vi "Set IConfiguration.vi"(8 "error in":errorcluster, 10 "IConfiguration":refnum<class "IConfiguration.lvclass">, 11 "Virtual Sensor from CSV in":refnum<class "Virtual Sensor from CSV.lvclass">) -> (0 "error out":errorcluster, 3 "Virtual Sensor from CSV out":refnum<class "Virtual Sensor from CSV.lvclass">)   [LabVIEW 2024, in "Virtual Sensor from CSV.lvclass"]
uses:
  Virtual Sensor from CSV.lvclass
  Interfaces/IConfiguration/IConfiguration.lvclass
  Virtual Sensor from CSV.lvclass/Virtual Sensor from CSV.ctl
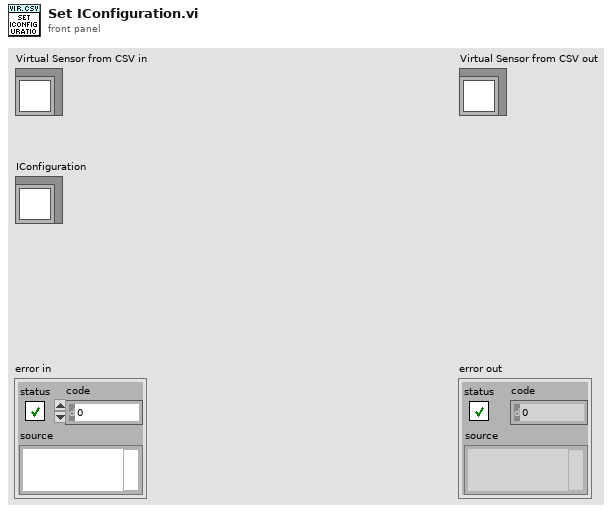
[diagram p1: front panel]
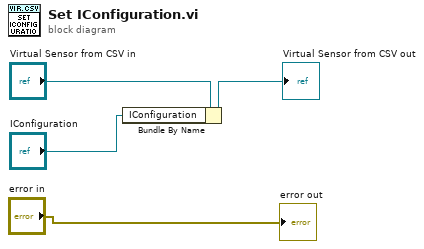
[diagram p0: block diagram]
diagram:
  n1 = Bundle By Name(cluster="Virtual Sensor from CSV in", "IConfiguration"="IConfiguration") -> (→"Virtual Sensor from CSV out":refnum<class "Virtual Sensor from CSV.lvclass">)
  "error out" <- "error in"
